vi "Test VI Analyzer Job.vi"() -> ()   [LabVIEW 2014]
uses:
  Core/LabVIEW CI Service/Extensions/VI Analyzer/VI Analyzer/VI Analyzer - STYP.ctl
  Core/LabVIEW CI Service/Classes/Status Updater/Status Updater.lvclass/Status Updater.ctl
  Core/LabVIEW CI Service/Classes/Job/Job.lvclass/Job.ctl
  Core/LabVIEW CI Service/Extensions/VI Analyzer/VI Analyzer/VI Analyzer.lvclass
  Core/LabVIEW CI Service/Classes/Status Updater/Status Updater.lvclass
  Core/LabVIEW CI Service/Classes/Job/Job.lvclass
panel:
  out "Results":T1 {"Status" items=["Service Error"=504, "Abort"=503, "Fail"=500, "Pass"=200]}
  out "Progress Percents":u32[](array[numeric])
  out "Steps":string[](array[string])
  in  "Executor Number":i32
  in  "Workspace Path":path=path "P:/alsmith/Sales/users/ACS/LabVIEW Continuous Integration/Test/VI Analyzer Job Test Code"
  in  "Test File":path=path "P:/alsmith/Sales/users/ACS/LabVIEW Continuous Integration/Jenkins Sample Project/Jenkins Sample Project.cfg"
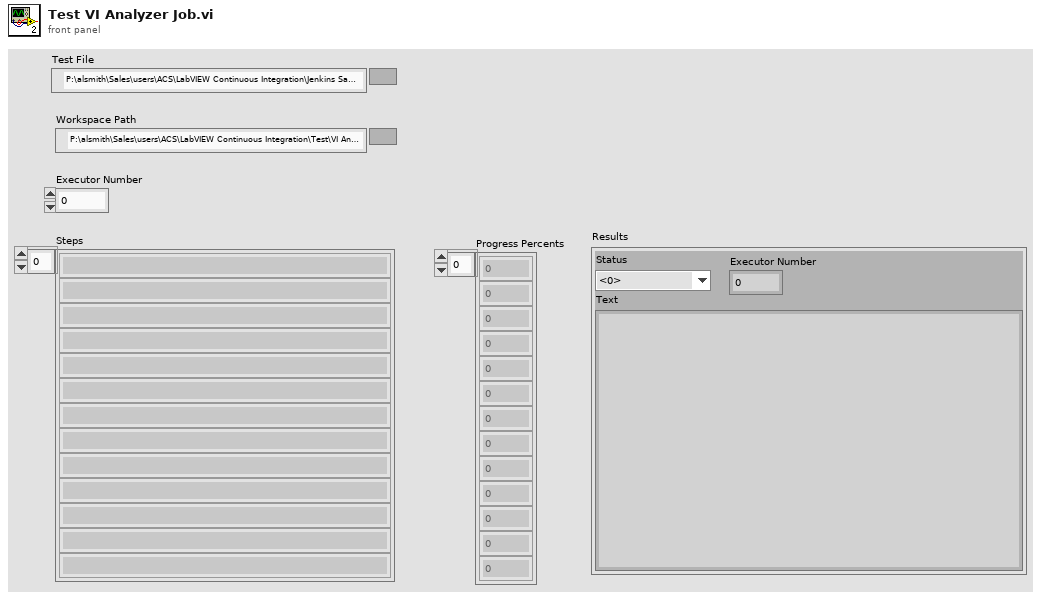
[diagram p1: front panel]
types:
  T1 = cluster{"Status":u16, "Text":string, "Executor Number":i32}
  T2 = typedef "VI Analyzer - STYP.ctl" = cluster{"Executor_Number":string, "Workspace_Path":string, "Test File":string}
  T3 = cluster{"Event Registration Refnum":refnum<event-registration>, "Event Registration Refnum":refnum<event-registration>}
  T4 = typedef "Job Results - STYP.ctl" = cluster{"Status":u16, "Text":string, "Executor Number":i32}
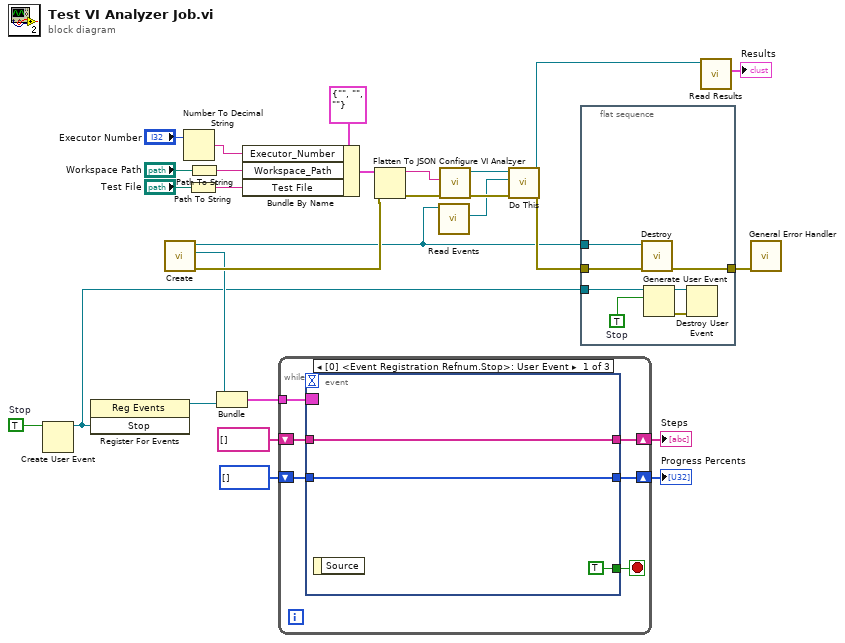
[diagram p0: block diagram]
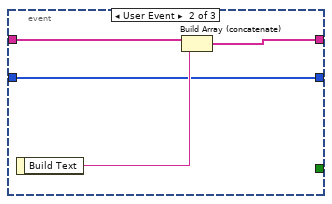
[diagram p2: hidden frame]
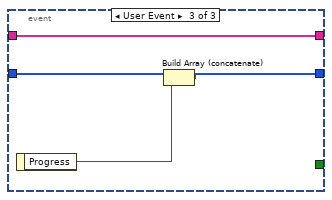
[diagram p3: hidden frame]
diagram:
  w13 = TRUE  # Stop
  n1 = Create User Event(user event datatype=w13) -> (user event=w9:refnum<user-event>)  [unwired: 1 in, 1 out]
  n2 = register-events(w9) -> (reference out=w10:refnum<event-registration>)  [unwired: 2 in, 1 out]
  n3 = call "Create.vi"() -> ("error out"=w15:errorcluster, "Event Registration Refnum"=w12:refnum<event-registration>, "Status Updater out"=w1:refnum<class "Status Updater.lvclass">)  [unwired: 9 in]
  n4 = Number To Decimal String(number="Executor Number") -> (decimal integer string=w25:string)  [unwired: 1 in]
  n5 = Path To String(path="Test File") -> (string=w26:string)
  n6 = Path To String(path="Workspace Path") -> (string=w21:string)
  n7 = Bundle("Event Registration Refnum"=w12, "Event Registration Refnum"=w10) -> (w11:T3)  [unwired: 1 in]
  n8 = Bundle By Name(cluster=T2 {"Executor_Number"="", "Workspace_Path"="", "Test File"=""} ("VI Analyzer - STYP.ctl"), "Executor_Number"=w25, "Workspace_Path"=w21, "Test File"=w26) -> (w28:T2)
  n9 = while {
    tunnel: w11 -> [w34]
    shift-right: [w31] -> w6
    shift-left: string[] [] -> [w32]
    shift-right: [w29] -> w5
    shift-left: u32[] [] -> [w30]
    stop <- w33 stop-if-true
    n10 = event shown="[0] <Event Registration Refnum.Stop>: User Event" {
      selector: w34 -> [_ _ _]
      dyn-events: _ -> [_ _ _]
      timeout: _ -> [_ _ _]
      tunnel: [TRUE _ _] -> w33
      tunnel: w32 -> [w36 w41 w45]
      tunnel: [w36 w40 w45] -> w31
      tunnel: w30 -> [w35 w38 w44]
      tunnel: [w35 w38 w43] -> w29
      event User Event {
        n11 = event-data() -> ()  [unwired: 1 in, 1 out]
      }
      event User Event {
        n12 = event-data() -> ("Build Text"=w39:string)  [unwired: 1 in]
        n13 = Build Array (concatenate)(w41, w39) -> (w40:string[])
      }
      event User Event {
        n14 = event-data() -> ("Progress"=w42:u32)  [unwired: 1 in]
        n15 = Build Array (concatenate)(w44, w42) -> (w43:u32[])
      }
    }
  }
  "Steps" <- w6
  "Progress Percents" <- w5
  n16 = Flatten To JSON(anything=w28, error in (no error)=w15) -> (JSON string=w24:string, 11:w23:errorcluster)  [unwired: 1 in]
  n17 = call "Read Events.vi"("Status Updater in"=w1) -> ("Status Events"=w16:refnum<class "Status Events.lvclass">)  [unwired: 10 in]
  n18 = call "Configure VI Analzyer.vi"("error in (no error)"=w23, "JSON String"=w24) -> ("error out"=w17:errorcluster, "VI Analyzer out"=w18:refnum<class "VI Analyzer.lvclass">)  [unwired: 8 in]
  n19 = call-dynamic "Do This.vi"("error in (no error)"=w17, "Status Events"=w16, "VI Analyzer in"=w18) -> ("error out"=w14:errorcluster, "VI Analyzer out"=w3:refnum<class "VI Analyzer.lvclass">)  [unwired: 7 in]
  n20 = flat-sequence {
    tunnel: w1 -> [w52]
    tunnel: w14 -> [w51]
    tunnel: w9 -> [w49]
    tunnel: [w48] -> w4
    frame #0 {
      w50 = TRUE  # Stop
      n21 = call "Destroy.vi"("error in (no error)"=w51, "Status Updater in"=w52) -> ("error out"=w48:errorcluster)  [unwired: 9 in]
      n22 = Generate User Event(user event=w49, event data cluster=w50) -> (user event out=w46:refnum<user-event>, error out=w47:errorcluster)  [unwired: 2 in]
      n23 = Destroy User Event(user event=w46, error in=w47) -> ()  [unwired: 1 out]
    }
  }
  n24 = call "Read Results.vi"("Job in"=w3) -> ("Results"=→"Results":T4)  [unwired: 10 in]
  n25 = call <vilib>:"General Error Handler.vi"("error in (no error)"=w4) -> ()  [unwired: 10 in, 5 out]
